vi "Yaw_with_complementary_filter.vi"(1 "ay":i32, 2 "ax":i32, 3 "*yaw":dbl) -> (0 "yaw":dbl)   [LabVIEW 2015]
doc: "yaw=atan2(ax,ay)*(180/pi)"
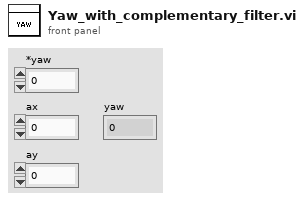
[diagram p1: front panel]
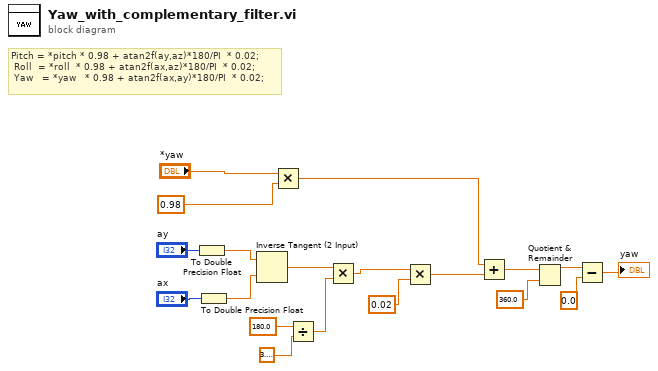
[diagram p0: block diagram]
diagram:
  # "Pitch = *pitch * 0.98 + atan2f(ay,az)*180/PI  * 0.02;\n Roll  = *roll  * 0.98 + atan2f(ax,az)*180/PI  * 0.02;\n Yaw   = *yaw   * 0.98 + atan2f(ax,ay)*180/PI  * 0.02;"
  n1 = To Double Precision Float(number="ay") -> (double precision float=w2:dbl)
  n2 = To Double Precision Float(number="ax") -> (double precision float=w1:dbl)
  n3 = Inverse Tangent (2 Input)(1:w1, 2:w2) -> (0:w19:dbl)
  n4 = Multiply(x="*yaw", y=0.98) -> (x*y=w9:dbl)
  n5 = Divide(x=180.0, y=3.141592653589793) -> (x/y=w16:dbl)
  n6 = Multiply(x=w19, y=w16) -> (x*y=w12:dbl)
  n7 = Multiply(x=w12, y=0.02) -> (x*y=w8:dbl)
  n8 = Add(x=w9, y=w8) -> (x+y=w7:dbl)
  n9 = Quotient & Remainder(x=w7, y=360.0) -> (x-y*floor(x/y)=w4:dbl)  [unwired: 1 out]
  n10 = Subtract(x=w4, y=0.0) -> (x-y=→"yaw":dbl)
